vi "Replay Movie.vi"() -> ()   [LabVIEW 2020]
panel:
  out "Codec Names":string[](array[string])
  out "Current folder":string
  in  "path":path=path "D:/dataToUpload"
  out "Total Frames":dbl
  in  "Stop":bool
  out "Preview":T1(plugin-control)
  out "Width":i32
  out "Height":i32
  out "Time Stamp (us)":u64
  out "Frame #":u64
  in  "No of Frame to Replay":i32=10000000
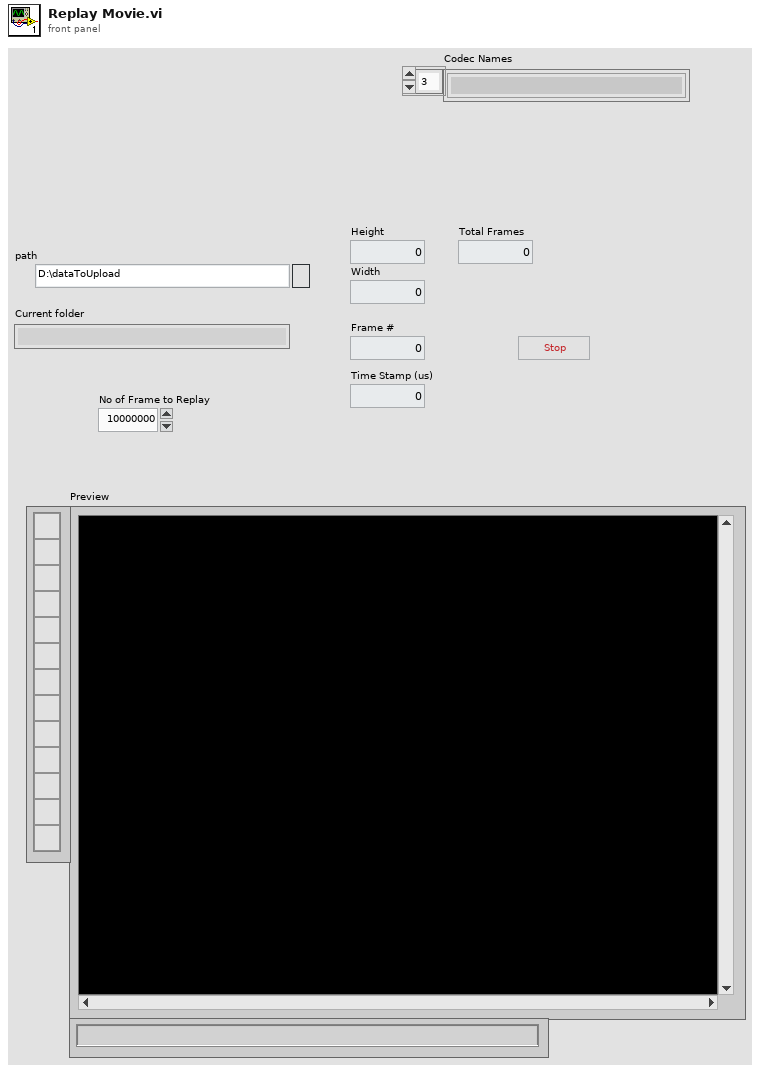
[diagram p1: front panel]
types:
  T1 = typedef "IMAQ Image.ctl" = refnum<image>
  T2 = enum16{"open", "replace", "create", "open or create", "replace or create", "replace or create with confirmation"}
  T3 = enum16{"big-endian, network order", "native, host order", "little-endian"}
  T4 = typedef "IMAQ AVI2 Refnum.ctl" = refnum<k20>
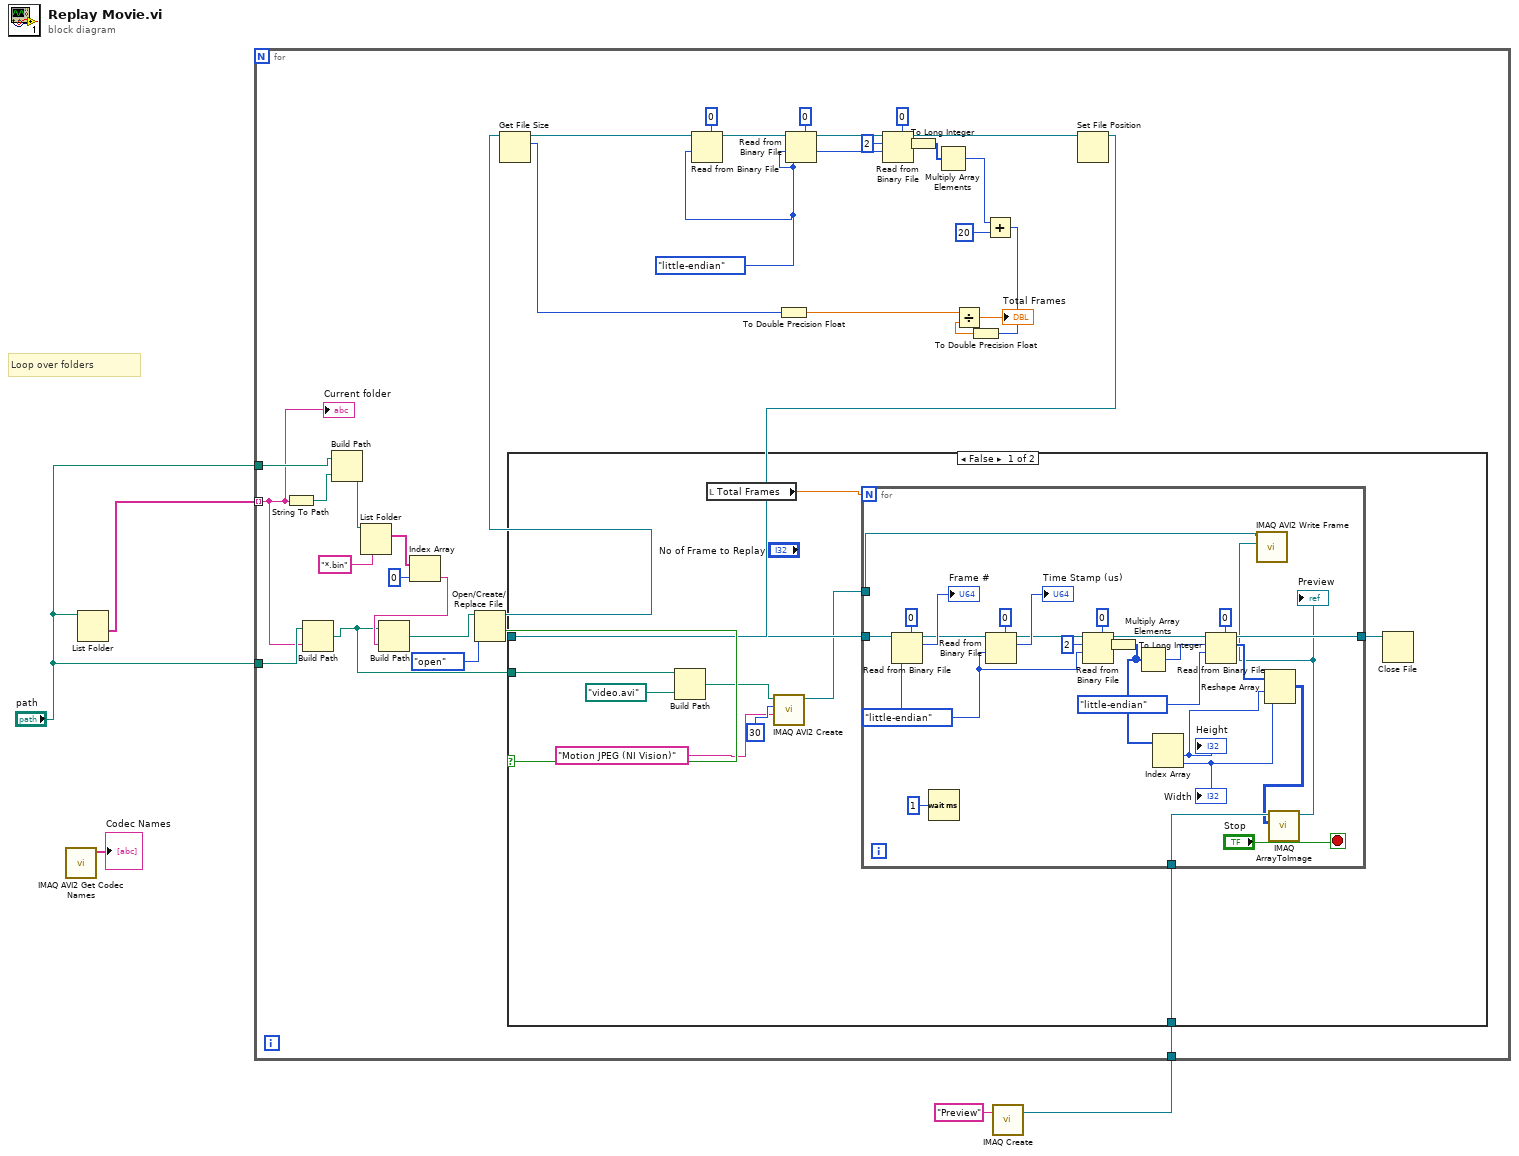
[diagram p0: block diagram]
diagram:
  # "Loop over folders"
  n1 = call "IMAQ AVI2 Get Codec Names"() -> ("Codec Names"=→"Codec Names":string[])  [unwired: 10 in, 1 out]
  n2 = List Folder(path="path") -> (folder names=w2:string[])  [unwired: 3 in, 3 out]
  n3 = call "IMAQ Create"("Image Name"="Preview") -> ("New Image"=w4:T1)  [unwired: 4 in, 1 out]
  n4 = for {
    tunnel: w4 -> [w37]
    tunnel: w2 -> [w6] mode=indexing
    tunnel: "path" -> [w11]
    tunnel: "path" -> [w10]
    w17 = T3."little-endian" ("byte order (0:big-endian, network order)")
    n5 = String To Path(string=w6) -> (path=w13:path)
    n6 = Build Path(base path=w10, name or relative path=w6) -> (appended path=w7:path)
    n7 = Build Path(base path=w11, name or relative path=w13) -> (appended path=w12:path)
    n8 = List Folder(path=w12, pattern="*.bin") -> (filenames=w15:string[])  [unwired: 2 in, 3 out]
    n9 = Index Array(array=w15, index=0) -> (element=w9:string)
    n10 = Build Path(base path=w7, name or relative path=w9) -> (appended path=w8:path)
    n11 = Open/Create/Replace File(file path (use dialog)=w8, operation (0:open)=T2."open") -> (refnum out=w25:refnum<file>, cancelled=w38:bool)  [unwired: 4 in, 1 out]
    n12 = Get File Size(file=w25) -> (refnum out=w24:refnum<file>, size (in bytes)=w22:i64)  [unwired: 1 in, 1 out]
    n13 = Read from Binary File(5:u64 0, 9:w17, 11:w24) -> (3:w31:refnum<file>)  [unwired: 3 in, 3 out]
    n14 = To Double Precision Float(number=w22) -> (double precision float=w20:dbl)
    n15 = Read from Binary File(5:u64 0, 9:w17, 11:w31) -> (3:w33:refnum<file>)  [unwired: 3 in, 3 out]
    n16 = Read from Binary File(5:u16 0, 9:w17, 10:2 ("count (1)"), 11:w33) -> (2:w35:u16[], 3:w26:refnum<file>)  [unwired: 2 in, 2 out]
    n17 = To Long Integer(number=w35) -> (32bit integer=w36:i32[])
    n18 = Multiply Array Elements(1:w36) -> (0:w28:i32)
    n19 = Add(x=w28, y=20) -> (x+y=w21:i32)
    n20 = To Double Precision Float(number=w21) -> (double precision float=w19:dbl)
    n21 = Divide(x=w20, y=w19) -> (x/y=→"Total Frames":dbl)
    n22 = Set File Position(refnum=w26) -> (refnum out=w23:refnum<file>)  [unwired: 3 in, 1 out]
    n23 = case shown="False" w38 {
      tunnel: w23 -> [w49 _]
      tunnel: w37 -> [w47 _]
      tunnel: w7 -> [w43 _]
      frame False {
        n24 = Build Path(base path=w43, name or relative path=path "video.avi" ("AVI Path")) -> (appended path=w42:path)
        n25 = local read "Total Frames"() -> (w41:dbl)
        n26 = call "IMAQ AVI2 Create"("Codec"="Motion JPEG (NI Vision)", "Frames Per Second"=u32 30, "AVI Path"=w42) -> ("AVI Refnum"=w45:T4)  [unwired: 7 in, 1 out]
        n27 = for {
          N: w41 -> [_]
          tunnel: w49 -> [w75]
          tunnel: [w61] -> w48
          tunnel: w47 -> [w60]
          tunnel: w45 -> [w50]
          stop <- "Stop" stop-if-true
          w53 = T3."little-endian" ("byte order (0:big-endian, network order)")
          n28 = Read from Binary File(5:u64 0, 9:w53, 11:w75) -> (2:→"Frame #":u64, 3:w70:refnum<file>)  [unwired: 3 in, 2 out]
          n29 = Wait (ms)(milliseconds to wait=u32 1) -> ()  [unwired: 1 out]
          n30 = Read from Binary File(5:u64 0, 9:w53, 11:w70) -> (2:→"Time Stamp (us)":u64, 3:w68:refnum<file>)  [unwired: 3 in, 2 out]
          n31 = Read from Binary File(5:u16 0, 9:w53, 10:2 ("count (1)"), 11:w68) -> (2:w63:u16[], 3:w64:refnum<file>)  [unwired: 2 in, 2 out]
          n32 = To Long Integer(number=w63) -> (32bit integer=w52:i32[])
          n33 = Multiply Array Elements(1:w52) -> (0:w65:i32)
          n34 = Index Array(array=w52) -> (element #1=w58:i32, element #2=w57:i32)  [unwired: 2 in]
          "Height" <- w58
          "Width" <- w57
          n35 = Read from Binary File(5:u8 0, 9:T3."little-endian" ("byte order (0:big-endian, network order)"), 10:w65, 11:w64) -> (2:w59:u8[], 3:w61:refnum<file>)  [unwired: 2 in, 2 out]
          n36 = Reshape Array(w59, w58, w57) -> (w56:u8[][])
          n37 = call "IMAQ ArrayToImage"("Image Pixels (U8)"=w56, "Image"=w60) -> ("Image Out"=w51:T1)  [unwired: 8 in, 1 out]
          "Preview" <- w51
          n38 = call "IMAQ AVI2 Write Frame"("Image"=w51, "AVI Refnum"=w50) -> ()  [unwired: 7 in, 3 out]
        }
        n39 = Close File(refnum=w48) -> ()  [unwired: 1 in, 2 out]
      }
      frame True {
      }
    }
    "Current folder" <- w6
  }
